vi "ConvertGP354OutputBytes.vi"(0 "Degas":bool, 1 "Enable Filament 1":bool, 2 "Enable Filament 2":bool, 3 "Medium Emission":bool, 4 "Ion Gauge":bool, 5 "High Emission":bool) -> (14 "Output Bytes":u8[](array[numeric]))   [LabVIEW 2011]
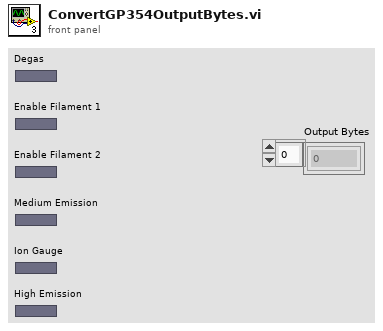
[diagram p1: front panel]
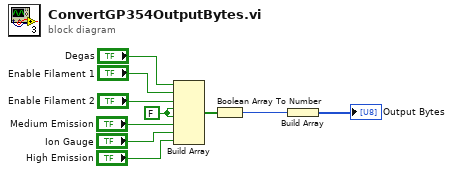
[diagram p0: block diagram]
diagram:
  w3 = FALSE
  n1 = Build Array("Degas", "Enable Filament 1", "Enable Filament 2", w3, w3, "Medium Emission", "Ion Gauge", "High Emission") -> (w6:bool[])
  n2 = Boolean Array To Number(Boolean array=w6) -> (number=w2:u8)
  n3 = Build Array(w2) -> (→"Output Bytes":u8[])
